vi "raspberry.vi"() -> ()   [LabVIEW 2015]
uses:
  <vilib>/MakerHub/LINX/Public/Peripherals/Digital/Digital Write 1 Chan.vi
  <vilib>/MakerHub/LINX/Public/Peripherals/Digital/Digital Write N Chans.vi
  <vilib>/MakerHub/LINX/Private/Local IO/LinxDigitalWrite.vi
  <vilib>/MakerHub/LINX/Public/Utilities/Check Channel.vi
  <vilib>/MakerHub/LINX/Public/Utilities/Open Serial.vi
  <vilib>/MakerHub/LINX/Private/Utilties/Generate Error.vi
  <vilib>/MakerHub/LINX/LMH-LINX.lvlib
panel:
  in  "Stop Button":bool
  in  "LED":bool
  in  "Raspberry Pin Numarasý":u8
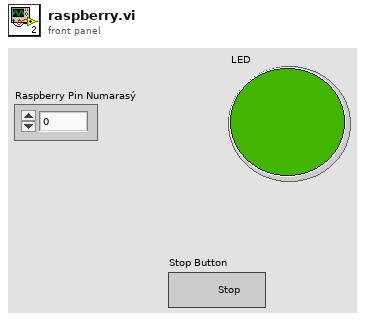
[diagram p1: front panel]
types:
  T1 = typedef "LMH-LINX.lvlib/LINX Ref.ctl" = cluster{"IO":T2, "Interface":T3, "LINX Device Config":T4}
  T2 = typedef "LMH-LINX.lvlib/Platform.ctl" = enum16{"Remote", "Local"}
  T3 = typedef "LMH-LINX.lvlib/Interface.ctl" = enum16{"Serial", "TCP"}
  T4 = typedef "LMH-LINX.lvlib/Device.lvlib/LINX Device Config.ctl" = cluster{"Interface":T3, "COM Port":refnum<visa-resource-name>, "TCP Configuration":T5, "Device Family":u8, "Device ID":u8, "Device Name":string, "TCP Ref":refnum<k5>, "Channels":T6}
  T5 = typedef "LMH-LINX.lvlib/Device.lvlib/TCP Config.ctl" = cluster{"IP Address":string, "Port":u16}
  T6 = typedef "LMH-LINX.lvlib/Channels.ctl" = cluster{"DI":u8[], "DO":u8[], "AI":u8[], "AO":u8[], "PWM":u8[], "QE":u8[], "UART":u8[], "I2C 2":u8[], "SPI":u8[], "CAN":u8[], "Servo":u8[], "AI Ref (V)":dbl, "AI Resolution (Bits)":u8, "AO Ref (V)":dbl, "AO Resolution (Bits)":u8}
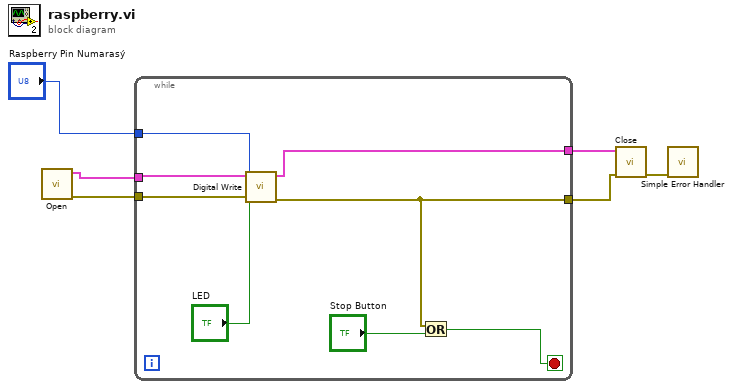
[diagram p0: block diagram]
diagram:
  n1 = call-poly <vilib>:"Open.vi"() -> ("Error Out"=w5:errorcluster, "LINX Resource"=w6:T1)  [unwired: 9 in, 1 out]
  n2 = while {
    tunnel: w6 -> [w14]
    tunnel: w5 -> [w13]
    tunnel: [w12] -> w4
    tunnel: [w8] -> w3
    tunnel: "Raspberry Pin Numarasý" -> [w11]
    stop <- w7 stop-if-true
    n3 = call-poly <vilib>:"Digital Write.vi"("Error In"=w13, "Output Value"="LED", "DO Channel"=w11, "LINX Resource"=w14) -> ("Error Out"=w8:errorcluster, "LINX Resource"=w12:T1)  [unwired: 6 in]
    n4 = Or(x=w8, y="Stop Button") -> (x .or. y?=w7:bool)
  }
  n5 = call <vilib>:"Close.vi"("Error In"=w3, "LINX Resource"=w4) -> ("Error Out"=w2:errorcluster)  [unwired: 9 in]
  n6 = call <vilib>:"Simple Error Handler.vi"("error in (no error)"=w2) -> ()  [unwired: 4 in, 5 out]
